vi "SerializeMessage.vi"(7 "MsgSerializer":refnum<class "MsgSerializer.lvclass">, 9 "error in (no error)":errorcluster, 10 "Value":variant, 11 "TestManagerMsg.Test in":refnum<class "TestManagerMsg.Test.lvclass">) -> (1 "error out":errorcluster, 3 "Serialized Message":string)   [LabVIEW 2020, in "Caraya.lvlib" / "TestManagerMsg.Test.lvclass"]
uses:
  TestManagerMsg.Test.lvclass
  MsgSerializer/MsgSerializer.lvclass
  Test Manager Message/TestManagerMsg.lvclass
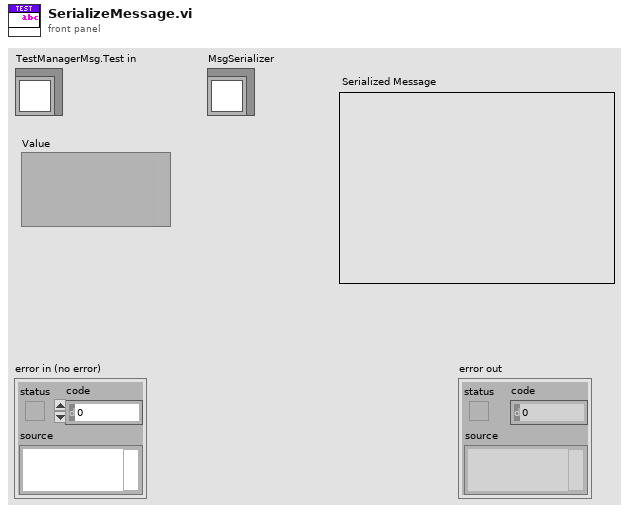
[diagram p1: front panel]
types:
  T1 = typedef "Caraya.lvlib/Test Result.lvclass/Test Registration Data.ctl" = cluster{"Name":string, "Call Chain":string[], "Time Stamp":timestamp, "Test ID":string, "Caller ID":string}
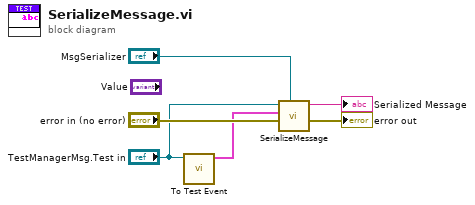
[diagram p0: block diagram]
diagram:
  n1 = call "To Test Event.vi"("TestManagerMsg.Test in"="TestManagerMsg.Test in") -> ("Test Registration"=w2:T1)  [unwired: 10 in]
  n2 = call-parent "SerializeMessage.vi"("MsgSerializer"="MsgSerializer", "error in (no error)"="error in (no error)", "Value"=w2, "TestManagerMsg in"="TestManagerMsg.Test in") -> ("error out"=→"error out":errorcluster, "Serialized Message"=→"Serialized Message":string)  [unwired: 6 in]
